vi "BoundsAbsoluteToRectangleSize.vi"(11 "RectangleAbsolute":T1) -> (3 "RectangleSize":T2)   [LabVIEW 2020, in "LcPictureBox.lvclass"]
uses:
  LcPictureBox.lvclass
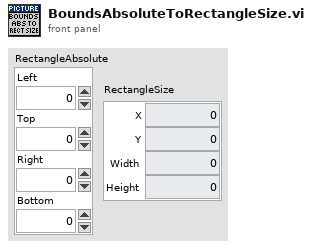
[diagram p1: front panel]
types:
  T1 = cluster{"Left":dbl, "Top":dbl, "Right":dbl, "Bottom":dbl}
  T2 = cluster{"X":sgl, "Y":sgl, "Width":sgl, "Height":sgl}
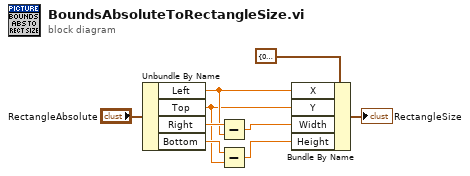
[diagram p0: block diagram]
diagram:
  n1 = Unbundle By Name("RectangleAbsolute") -> ("Left"=w5:dbl, "Top"=w2:dbl, "Right"=w6:dbl, "Bottom"=w3:dbl)
  n2 = Subtract(x=w6, y=w5) -> (x-y=w4:dbl)
  n3 = Subtract(x=w3, y=w2) -> (x-y=w1:dbl)
  n4 = Bundle By Name(cluster=T2 {"X"=0.0, "Y"=0.0, "Width"=0.0, "Height"=0.0} ("RectangleSize"), "X"=w5, "Y"=w2, "Width"=w4, "Height"=w1) -> (→"RectangleSize":T2)
